vi "M-227 Timeout Check.vi"(0 "Action":T1, 2 "User Input?":bool) -> (8 "Timeout?":bool, 15 "Action (Dup)":T1)   [LabVIEW 2016]
uses:
  Stages Controls/Stage Actions.ctl
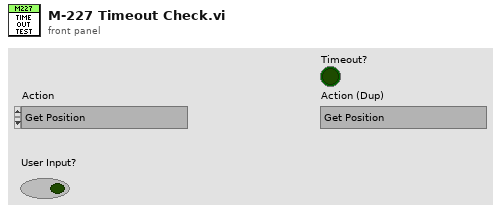
[diagram p1: front panel]
types:
  T1 = typedef "Stage Actions.ctl" = enum16{"Get Position", "MVR", "MOVE", "HALT", "ONTARGET", "ERROR", "REFERENCE", "INIT", "VELOCITY", "STATUS", "EXIT", "HOME", "ZEROPOS", "NANOPOS", "ANALOG", "QUIT"}
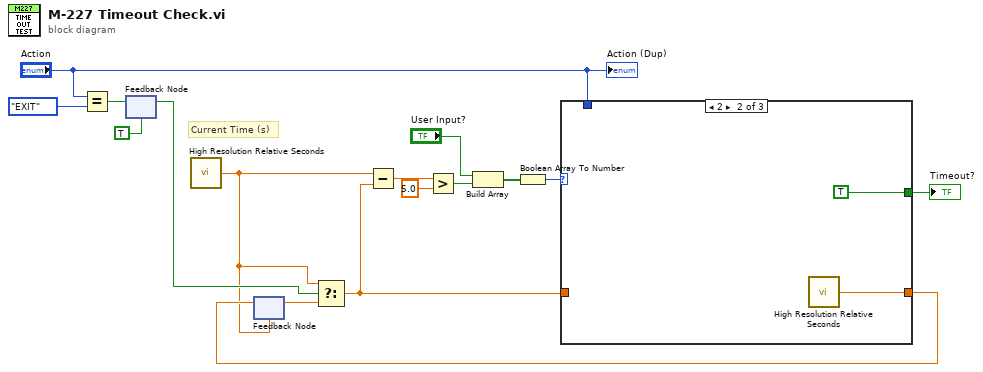
[diagram p0: block diagram]
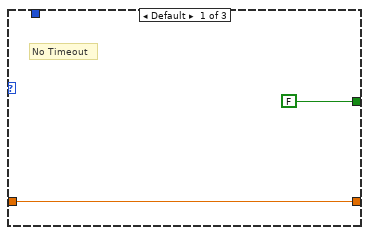
[diagram p2: hidden frame]
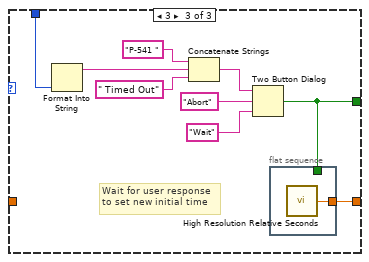
[diagram p3: hidden frame]
diagram:
  # "Current Time (s)"
  n1 = Equal?(x="Action", y=Stage_Actions."EXIT") -> (x = y?=w6:bool)
  n2 = feedback-in #1(w6) -> ()
  n3 = feedback #1(TRUE) -> (w2:bool)
  n4 = call <vilib>:"High Resolution Relative Seconds.vi"() -> ("relative seconds"=w1:dbl)
  n5 = feedback #2(w1) -> (w4:dbl)
  n6 = Select(t=w1, s=w2, f=w4) -> (s? t:f=w3:dbl)
  n7 = Subtract(x=w1, y=w3) -> (x-y=w16:dbl)
  n8 = Greater?(x=w16, y=5.0) -> (0:w13:bool)
  n9 = Build Array("User Input?", w13) -> (w12:bool[])
  n10 = Boolean Array To Number(Boolean array=w12) -> (number=w11:u32)
  n11 = case shown="2" w11 {
    tunnel: [FALSE ("T button?") TRUE ("T button?") w21] -> w10
    tunnel: "Action" -> [_ _ w24]
    tunnel: w3 -> [w17 _ _]
    tunnel: [w17 w19 w22] -> w5
    frame Default {
      # "No Timeout"
    }
    frame 2 {
      n12 = call <vilib>:"High Resolution Relative Seconds.vi"() -> ("relative seconds"=w19:dbl)
    }
    frame 3 {
      # "Wait for user response\nto set new initial time"
      n13 = Format Into String(w24) -> (resulting string=w29:string)  [unwired: 3 in, 1 out]
      n14 = Concatenate Strings("P-541 " ("string"), w29, " Timed Out" ("message")) -> (w28:string)
      n15 = Two Button Dialog(message=w28, 1:"Wait" ("F button name (\"Cancel\")"), 2:"Abort" ("T button name (\"OK\")")) -> (T button?=w21:bool)
      n16 = flat-sequence {
        tunnel: [w30] -> w22
        tunnel: w21 -> [_]
        frame #0 {
          n17 = call <vilib>:"High Resolution Relative Seconds.vi"() -> ("relative seconds"=w30:dbl)
        }
      }
    }
  }
  "Timeout?" <- w10
  n18 = feedback-in #2(w5) -> ()
  "Action (Dup)" <- "Action"
